vi "ReadCoordinates.vi"(11 "Ctl Refnum":refnum<vi>) -> (3 "appended array":i32[](array[numeric]))   [LabVIEW 2017]
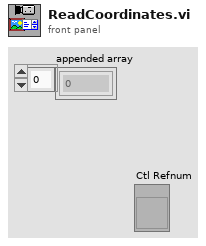
[diagram p1: front panel]
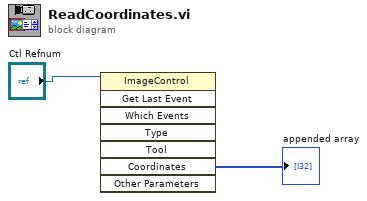
[diagram p0: block diagram]
diagram:
  n1 = invoke class="ImageControl" method="Get Last Event"(reference="Ctl Refnum") -> ("Coordinates"=→"appended array":i32[])  [unwired: 7 in, 7 out]
